vi "MSEncoder SubVI AddScanIndex.vi"(7 "xml string":string, 8 "error in (no error)":errorcluster, 11 "Refnum in":refnum<k34>) -> (0 "error out":errorcluster, 1 "Index":i32, 3 "Refnum out":refnum<k34>)   [LabVIEW 2018, in "MSEncoder.lvclass"]
uses:
  MSEncoder.lvclass
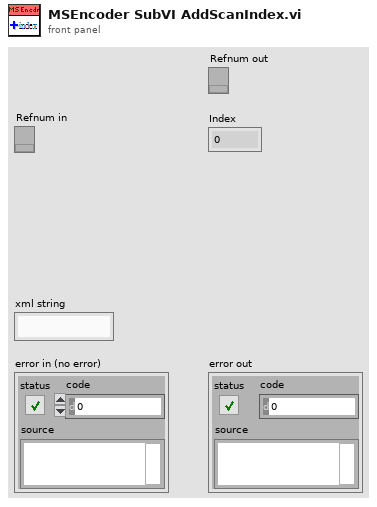
[diagram p1: front panel]
types:
  T1 = enum16{"open", "open or create", "create or replace", "create", "open (read-only)"}
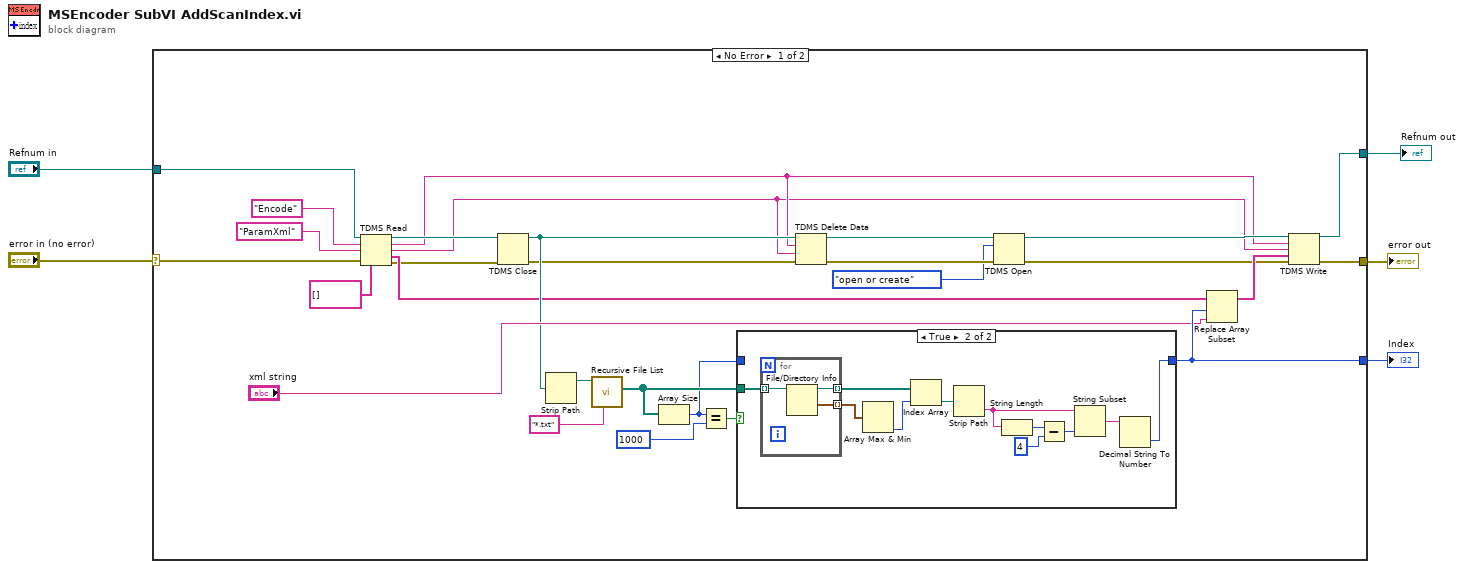
[diagram p0: block diagram]
diagram:
  n1 = case shown="No Error" "error in (no error)" {
    selector: "error in (no error)" -> [w7 w50]
    tunnel: [w33 _] -> w5
    tunnel: [w23 w50] -> w4
    tunnel: [w16 w49] -> w3
    tunnel: "Refnum in" -> [w6 w49]
    frame No Error {
      n2 = TDMS Read(0:w6, 5:"Encode" ("group name in (Untitled)"), 7:"ParamXml" ("channel name(s) in (Untitled)"), 11:w7, 12:string[] []) -> (4:w12:refnum<k34>, 6:w11:string, 8:w10:string, 10:w9:string[], 15:w8:errorcluster)  [unwired: 3 in, 1 out]
      n3 = TDMS Close(8:w8, 11:w12) -> (0:w20:errorcluster, 3:w25:path)
      n4 = Strip Path(path=w25) -> (stripped path=w26:path)  [unwired: 1 out]
      n5 = call <vilib>:"Recursive File List.vi"("pattern"="*.txt", "Folder Path"=w26) -> ("All Files in Dir"=w32:path[])  [unwired: 5 in, 4 out]
      n6 = Array Size(array=w32) -> (size(s)=w30:i32)
      n7 = Equal?(x=w30, y=1000) -> (x = y?=w29:bool)
      n8 = case shown="True" w29 {
        tunnel: w30 -> [w34 _]
        tunnel: [w34 w39] -> w33
        tunnel: w32 -> [_ w38]
        frame False {
        }
        frame True {
          n9 = for {
            tunnel: w38 -> [w48] mode=indexing
            tunnel: [w47] -> w37 mode=indexing
            tunnel: [w46] -> w36 mode=indexing
            n10 = File/Directory Info(path=w48) -> (path out=w46:path, last mod=w47:timestamp)  [unwired: 1 in, 5 out]
          }
          n11 = Array Max & Min(array=w37) -> (min index (indices)=w35:i32)  [unwired: 3 out]
          n12 = Index Array(array=w36, index=w35) -> (element=w45:path)
          n13 = Strip Path(path=w45) -> (name=w44:string)  [unwired: 1 out]
          n14 = String Length(string=w44) -> (length=w43:i32)
          n15 = Subtract(x=w43, y=4) -> (x-y=w41:i32)
          n16 = String Subset(string=w44, length (rest)=w41) -> (substring=w40:string)  [unwired: 1 in]
          n17 = Decimal String To Number(string=w40) -> (number=w39:i32)  [unwired: 2 in, 1 out]
        }
      }
      n18 = TDMS Delete Data(8:w20, 9:w10, 10:w11, 11:w25) -> (0:w21:errorcluster, 3:w17:path)  [unwired: 3 in]
      n19 = TDMS Open(8:w21, 10:T1."open or create" ("operation (0:open)"), 11:w17) -> (0:w22:errorcluster, 3:w18:refnum<k34>)  [unwired: 4 in]
      n20 = Replace Array Subset(array=w9, new element="xml string", index=w33) -> (w24:string[])
      n21 = TDMS Write(0:w18, 5:w11, 7:w10, 9:w24, 11:w22) -> (4:w16:refnum<k34>, 15:w23:errorcluster)  [unwired: 1 in, 2 out]
    }
    frame Error {
    }
  }
  "Index" <- w5
  "error out" <- w4
  "Refnum out" <- w3
